vi "create_image.vi"(8 "error in":errorcluster, 10 "Enum in":refnum<vi>, 11 "base path":path) -> (0 "error out":errorcluster, 3 "path":path)   [LabVIEW 2018]
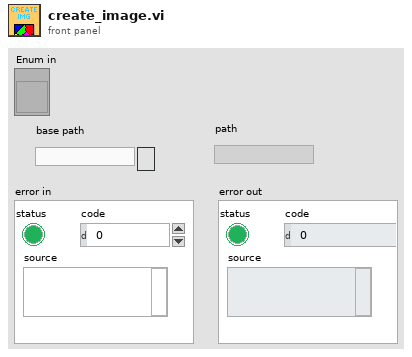
[diagram p1: front panel]
types:
  T1 = enum16{"open", "replace", "create", "open or create", "replace or create", "replace or create with confirmation"}
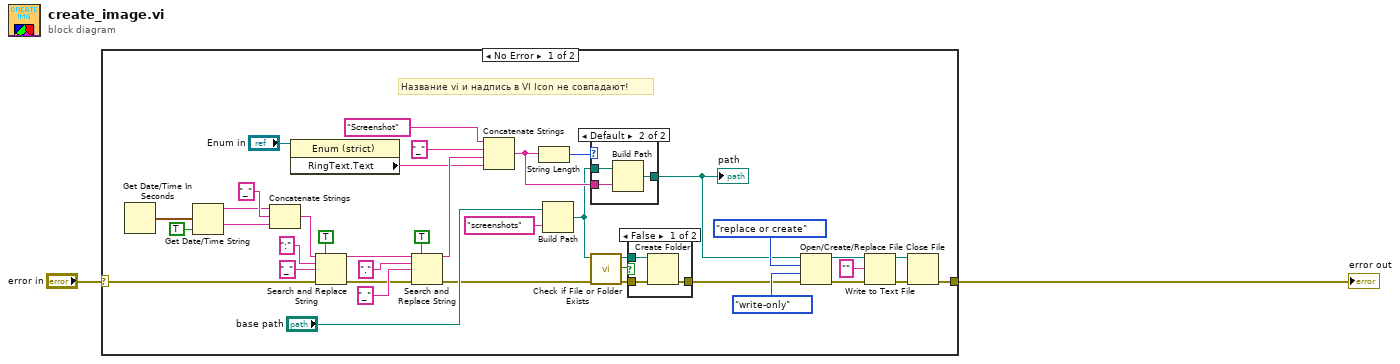
[diagram p0: block diagram]
diagram:
  n1 = case shown="No Error" "error in" {
    selector: "error in" -> [w6 w50]
    tunnel: [w14 w50] -> w2
    frame No Error {
      # "Название vi и надпись в VI Icon не совпадают!"
      n2 = Get Date/Time In Seconds() -> (seconds since 1Jan1904=w20:timestamp)
      n3 = Get Date/Time String(seconds (now)=w20, want seconds? (F)=TRUE) -> (date string=w21:string, time string=w29:string)  [unwired: 1 in]
      n4 = Concatenate Strings(w21, "_" ("string"), w29) -> (w22:string)
      n5 = property class="Enum (strict)"(reference="Enum in") -> ("RingText.Text"=w3:string)  [unwired: 1 in, 2 out]
      n6 = Search and Replace String(replace all?=TRUE, input string=w22, search string=":", replace string="_" ("replace string (\"\")"), error in=w6) -> (result string=w25:string, error out=w10:errorcluster)  [unwired: 3 in, 2 out]
      n7 = Search and Replace String(replace all?=TRUE, input string=w25, search string=".", replace string="_" ("replace string (\"\")"), error in=w10) -> (result string=w17:string, error out=w8:errorcluster)  [unwired: 3 in, 2 out]
      n8 = Concatenate Strings("Screenshot" ("name or relative path"), "_" ("name or relative path"), w17, w3) -> (w33:string)
      n9 = String Length(string=w33) -> (length=w32:i32)
      n10 = Build Path(base path="base path", name or relative path="screenshots") -> (appended path=w13:path)
      n11 = case shown="Default" w32 {
        tunnel: [w46 w49] -> w15
        tunnel: w13 -> [w46 w48]
        tunnel: w33 -> [_ w47]
        frame 0 {
        }
        frame Default {
          n12 = Build Path(base path=w48, name or relative path=w47) -> (appended path=w49:path)
        }
      }
      "path" <- w15
      n13 = call <vilib>:"Check if File or Folder Exists.vi"("error in (no error)"=w8, "path"=w13) -> ("error out"=w7:errorcluster, "file or folder exists?"=w12:bool, "dup path"=w11:path)  [unwired: 7 in]
      n14 = case shown="False" w12 {
        tunnel: w11 -> [w44 _]
        tunnel: w7 -> [w43 w45]
        tunnel: [w42 w45] -> w9
        frame False {
          n15 = Create Folder(path (use dialog)=w44, error in=w43) -> (error out=w42:errorcluster)  [unwired: 1 in, 2 out]
        }
        frame True {
        }
      }
      n16 = Open/Create/Replace File(file path (use dialog)=w15, error in=w9, operation (0:open)=T1."replace or create", access (0:read/write)=enum16{"read/write", "read-only", "write-only"}."write-only") -> (refnum out=w39:refnum<file>, error out=w40:errorcluster)  [unwired: 2 in, 1 out]
      n17 = Write to Text File(file (use dialog)=w39, text="", error in=w40) -> (refnum out=w38:refnum<file>, error out=w37:errorcluster)  [unwired: 1 in, 1 out]
      n18 = Close File(refnum=w38, error in=w37) -> (error out=w14:errorcluster)  [unwired: 1 out]
    }
    frame Error {
    }
  }
  "error out" <- w2
